vi "Create from VI.vi"(8 "error in (no error)":errorcluster, 9 "Test Method VI Path":path, 10 "Test Case LVCLass Path":path) -> (0 "error out":errorcluster, 3 "LUnit Test Case V2 out":refnum<class "LUnit Test Case V2.lvclass">)   [LabVIEW 2020, in "LUnit Test Case V2.lvclass"]
uses:
  LUnit Test Case V2.lvclass
  LUnit Test Case V2.lvclass/LUnit Test Case V2.ctl
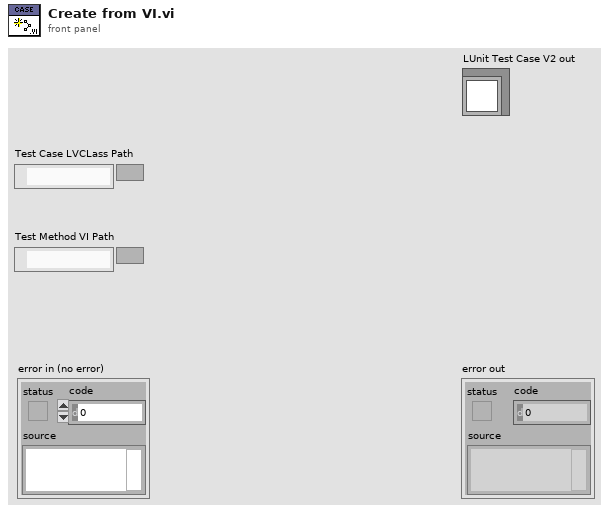
[diagram p1: front panel]
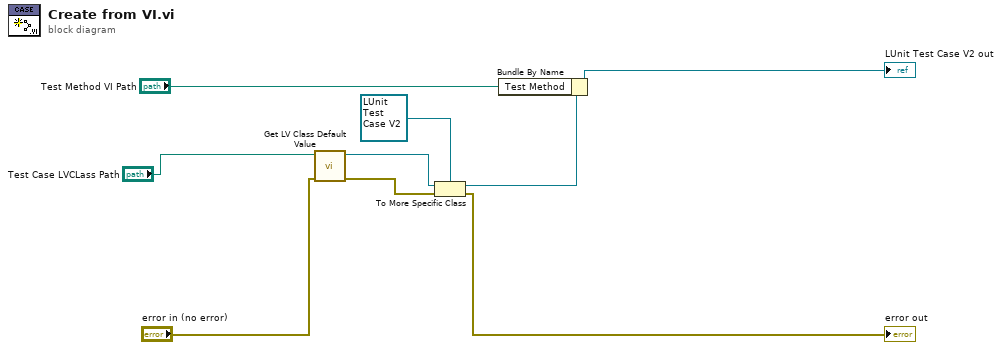
[diagram p0: block diagram]
diagram:
  n1 = call <vilib>:"Get LV Class Default Value.vi"("error in (no error)"="error in (no error)", "class path"="Test Case LVCLass Path") -> ("error out"=w4:errorcluster, "object"=w5:refnum<class>)  [unwired: 8 in]
  n2 = To More Specific Class(target class=refnum<class "LUnit Test Case V2.lvclass"> refnum ("LUnit Test Case V2.lvclass"), reference=w5, error in=w4) -> (specific class reference=w6:refnum<class "LUnit Test Case V2.lvclass">, error out=→"error out":errorcluster)
  n3 = Bundle By Name(cluster=w6, "Test Method"="Test Method VI Path") -> (→"LUnit Test Case V2 out":refnum<class "LUnit Test Case V2.lvclass">)
